vi "setSerializedData.vi"(0 "reference":refnum<class "StateTransitionEdge.lvclass">, 1 "startNode":refnum<class "AbstractNode.lvclass">, 2 "endNode":refnum<class "AbstractNode.lvclass">, 3 "xmlOut":string, 5 "error in (no error)":errorcluster) -> (14 "reference out":refnum<class "StateTransitionEdge.lvclass">, 19 "error out":errorcluster)   [LabVIEW 2014, in "StateTransitionEdge.lvclass"]
doc: "setSerializedData"
uses:
  <resource>/Framework/Providers/Open_GDS/UML/StateTransitionEdge_class/StateTransitionEdge.lvclass
  <resource>/Framework/Providers/Open_GDS/UML/AbstractNode_class/AbstractNode.lvclass
  <resource>/Framework/Providers/Open_GDS/UML/AbstractNode_class/ObjectReference.ctl
  <resource>/Framework/Providers/Open_GDS/UML/LineStyle_class/ObjectReference.ctl
  <resource>/Framework/Providers/Open_GDS/UML/ArrowHead_class/ObjectReference.ctl
  <resource>/Framework/Providers/Open_GDS/UML/General/Point/Point Point2D.ctl
  <resource>/Framework/Providers/Open_GDS/UML/BentStyle_class/ObjectReference.ctl
  <resource>/Framework/Providers/Open_GDS/UML/ReversedEngineering/ReversedEngineering_ViDependencyDetailsType.ctl
  <resource>/Framework/Providers/Open_GDS/UML/LineStyle_class/LineStyleType.ctl
  <resource>/Framework/Providers/Open_GDS/UML/ArrowHead_class/ArrowHeadType.ctl
  <resource>/Framework/Providers/Open_GDS/UML/LineStyle_class/LineStyle.lvclass
  <resource>/Framework/Providers/Open_GDS/UML/ArrowHead_class/ArrowHead.lvclass
  <resource>/Framework/Providers/Open_GDS/UML/BentStyle_class/BentStyle.lvclass
  <resource>/Framework/Providers/Open_GDS/UML/ClassRelationshipEdge_class/ClassRelationshipEdge.lvclass
  <resource>/Framework/Providers/Open_GDS/UML/SegmentedLineEdge_class/SegmentedLineEdge.lvclass
  <resource>/Framework/Providers/Open_GDS/UML/AbstractEdge_class/AbstractEdge.lvclass
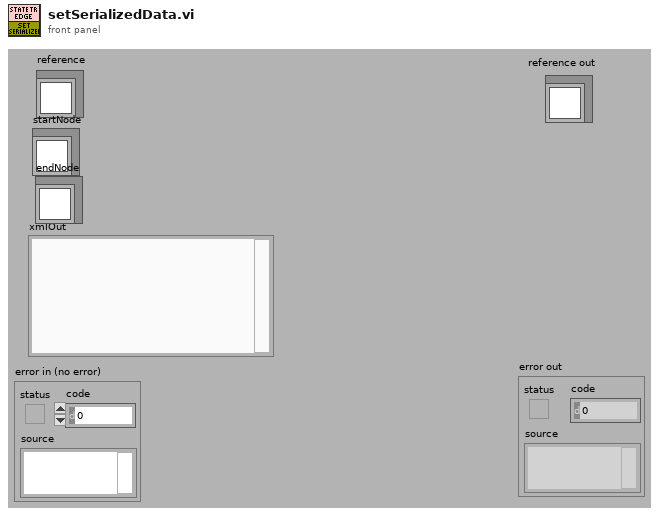
[diagram p1: front panel]
types:
  T1 = typedef "LineStyle.lvclass/ObjectReference.ctl" = refnum<k1>
  T2 = typedef "ArrowHead.lvclass/ObjectReference.ctl" = refnum<k1>
  T3 = typedef "Point Point2D.ctl" = cluster{"x":dbl, "y":dbl}
  T4 = typedef "BentStyle.lvclass/ObjectReference.ctl" = refnum<k1>
  T5 = typedef "ReversedEngineering_ViDependencyDetailsType.ctl" = cluster{"ThisVIs/Ctls":path[], "Dependent_VIs/Ctls":path[]}
  T6 = typedef "AbstractNode.lvclass/ObjectReference.ctl" = refnum<k1>
  T7 = cluster{"Base class":cluster{"Base class":cluster{"Base class":cluster{"Base class":cluster{"start":T6, "end":T6}}, "lineStyle":T1, "startArrowHead":T2, "endArrowHead":T2, "startLabel":string, "midLabel":string, "endLabel":string, "MidLabelOffset":T3, "SplitWire":bool}, "bentStyleRef":T4, "startConnectionOffset":cluster{"x":i32, "y":i32}, "endConnectionOffset":cluster{"x":i32, "y":i32}, "MidLineOffset":cluster{"x":i32, "y":i32}, "DepClass":T5}, "angle":dbl}
  T8 = typedef "LineStyle.lvclass/LineStyleType.ctl" = enum16{"SOLID", "DOTTED"}
  T9 = typedef "ArrowHead.lvclass/ArrowHeadType.ctl" = enum16{"NONE", "TRIANGLE", "BLACK_TRIANGLE", "V", "HALF_V", "DIAMOND", "BLACK_DIAMOND"}
  T10 = cluster{"Attributes":cluster{"Base class":cluster{"Base class":cluster{"Base class":cluster{"Base class":cluster{"start":T6, "end":T6}}, "lineStyle":T1, "startArrowHead":T2, "endArrowHead":T2, "startLabel":string, "midLabel":string, "endLabel":string, "MidLabelOffset":T3, "SplitWire":bool}, "bentStyleRef":T4, "startConnectionOffset":cluster{"x":i32, "y":i32}, "endConnectionOffset":cluster{"x":i32, "y":i32}, "MidLineOffset":cluster{"x":i32, "y":i32}, "DepClass":T5}, "angle":dbl}, string, string, string}
  T11 = typedef "SegmentedLineEdge.lvclass/ObjectAttributes.ctl" = cluster{"lineStyle":refnum<class "LineStyle.lvclass">, "startArrowHead":refnum<class "ArrowHead.lvclass">, "endArrowHead":refnum<class "ArrowHead.lvclass">, "startLabel":string, "midLabel":string, "endLabel":string, "MidLabelOffset":T3, "SplitWire":bool}
  T12 = typedef "AbstractEdge.lvclass/ObjectAttributes.ctl" = cluster{"start":refnum<class "AbstractNode.lvclass">, "end":refnum<class "AbstractNode.lvclass">}
  T13 = typedef "StateTransitionEdge.lvclass/ObjectAttributes.ctl" = cluster{"angle":dbl}
  T14 = typedef "ClassRelationshipEdge.lvclass/ObjectAttributes.ctl" = cluster{"bentStyleRef":refnum<class "BentStyle.lvclass">, "startConnectionOffset":cluster{"x":i32, "y":i32}, "endConnectionOffset":cluster{"x":i32, "y":i32}, "MidLineOffset":cluster{"x":i32, "y":i32}, "DepClass":T5}
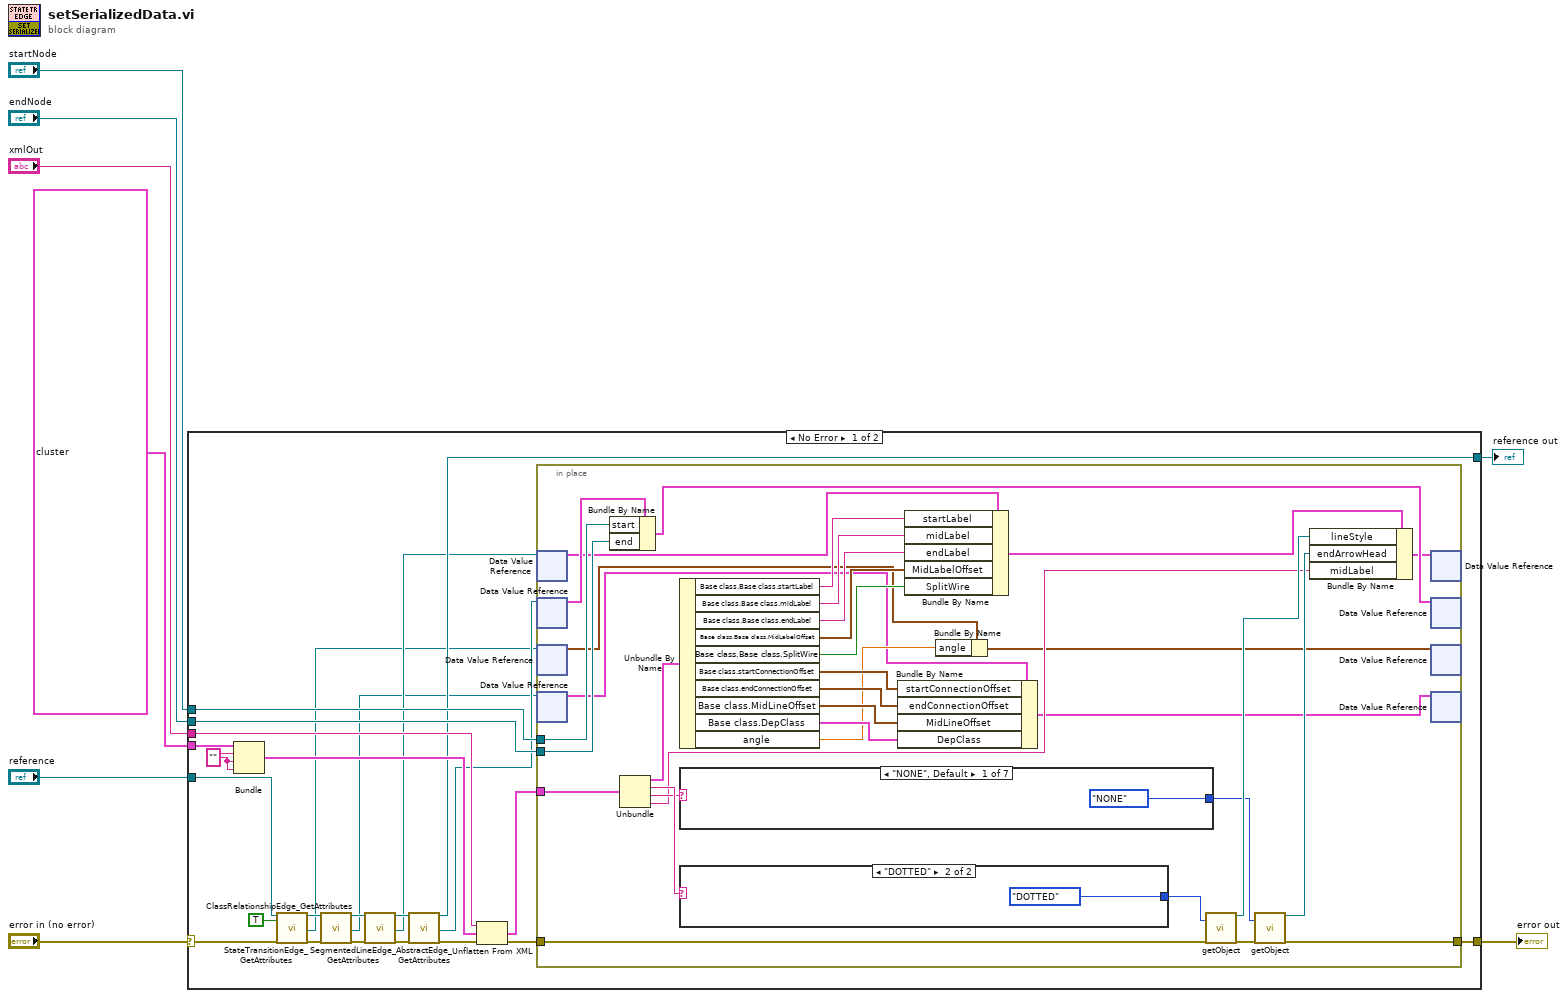
[diagram p0: block diagram]
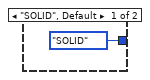
[diagram p2: hidden frame]
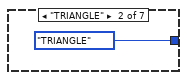
[diagram p3: hidden frame]
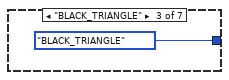
[diagram p4: hidden frame]
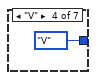
[diagram p5: hidden frame]
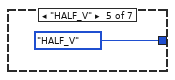
[diagram p6: hidden frame]
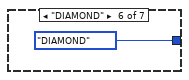
[diagram p7: hidden frame]
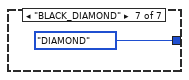
[diagram p8: hidden frame]
diagram:
  n1 = case shown="No Error" "error in (no error)" {
    selector: "error in (no error)" -> [w31 w75]
    tunnel: "reference" -> [w32 w76]
    tunnel: [w13 w76] -> w6
    tunnel: [w30 w75] -> w5
    tunnel: "xmlOut" -> [w19 _]
    tunnel: "startNode" -> [w29 _]
    tunnel: "endNode" -> [w28 _]
    tunnel: T7 {"Base class"={"Base class"={"Base class"={"Base class"={"start"=refnum, "end"=refnum}}, "lineStyle"=refnum, "startArrowHead"=refnum, "endArrowHead"=refnum, "startLabel"="", "midLabel"="", "endLabel"="", "MidLabelOffset"={"x"=0.0, "y"=0.0}, "SplitWire"=FALSE}, "bentStyleRef"=refnum, "startConnectionOffset"={"x"=0, "y"=0}, "endConnectionOffset"={"x"=0, "y"=0}, "MidLineOffset"={"x"=0, "y"=0}, "DepClass"={"ThisVIs/Ctls"=[], "Dependent_VIs/Ctls"=[]}}, "angle"=0.0} ("Attributes") -> [w26 _]
    frame No Error {
      w27 = ""
      n2 = Bundle("Attributes"=w26, w27, w27, w27) -> (w17:T10)  [unwired: 1 out]
      n3 = call <resource>:"StateTransitionEdge_GetAttributes.vi"("reference in"=w32, "OnlyGetDvrReference(False)"=TRUE, "error in (no error)"=w31) -> ("reference out"=w24:refnum<class "StateTransitionEdge.lvclass">, "DataRef"=w9:refnum<data-value>, "error out"=w23:errorcluster)  [unwired: 13 in, 1 out]
      n4 = call <resource>:"ClassRelationshipEdge_GetAttributes.vi"("reference in"=w24, "error in (no error)"=w23) -> ("reference out"=w22:refnum<class "StateTransitionEdge.lvclass">, "DataRef"=w10:refnum<data-value>, "error out"=w21:errorcluster)  [unwired: 14 in, 1 out]
      n5 = call <resource>:"SegmentedLineEdge_GetAttributes.vi"("reference in"=w22, "error in (no error)"=w21) -> ("reference out"=w16:refnum<class "StateTransitionEdge.lvclass">, "DataRef"=w11:refnum<data-value>, "error out"=w15:errorcluster)  [unwired: 14 in, 1 out]
      n6 = call <resource>:"AbstractEdge_GetAttributes.vi"("reference in"=w16, "error in (no error)"=w15) -> ("reference out"=w13:refnum<class "StateTransitionEdge.lvclass">, "DataRef"=w12:refnum<data-value>, "error out"=w14:errorcluster)  [unwired: 14 in, 1 out]
      n7 = Unflatten From XML(xml string=w19, type=w17, error in (no error)=w14) -> (value=w20:T10, error out=w18:errorcluster)
      n8 = in-place {
        in-place-border: [w63] -> w30
        in-place-border: w29 -> [w43]
        in-place-border: w28 -> [w42]
        in-place-border: w20 -> [w59]
        in-place-border: w18 -> [w58]
        n9 = in-place-dvr #1(w11) -> (w39:T11)  [unwired: 1 out]
        n10 = in-place-dvr #2(w12) -> (w41:T12)  [unwired: 1 out]
        n11 = in-place-dvr #3(w9) -> (w35:T13)  [unwired: 1 out]
        n12 = in-place-dvr #4(w10) -> (w36:T14)  [unwired: 1 out]
        n13 = Bundle By Name(cluster=w41, "start"=w43, "end"=w42) -> (w40:T12)
        n14 = Unbundle(w59) -> ("Attributes"=w47:T7, w46:string, w45:string, w44:string)
        n15 = Unbundle By Name(w47) -> ("Base class.Base class.startLabel"=w57:string, "Base class.Base class.midLabel"=w56:string, "Base class.Base class.endLabel"=w55:string, "Base class.Base class.MidLabelOffset"=w54:T3, "Base class.Base class.SplitWire"=w53:bool, "Base class.startConnectionOffset"=w52:cluster{"x":i32, "y":i32}, "Base class.endConnectionOffset"=w51:cluster{"x":i32, "y":i32}, "Base class.MidLineOffset"=w50:cluster{"x":i32, "y":i32}, "Base class.DepClass"=w49:T5, "angle"=w48:dbl)
        n16 = case shown="\"NONE\", Default" w45 {
          tunnel: [ArrowHeadType."NONE" ("arrowHead") ArrowHeadType."TRIANGLE" ("arrowHead") ArrowHeadType."BLACK_TRIANGLE" ("arrowHead") ArrowHeadType."V" ("arrowHead") ArrowHeadType."HALF_V" ("arrowHead") ArrowHeadType."DIAMOND" ("arrowHead") ArrowHeadType."DIAMOND" ("arrowHead")] -> w62
          frame "NONE", Default {
          }
          frame "TRIANGLE" {
          }
          frame "BLACK_TRIANGLE" {
          }
          frame "V" {
          }
          frame "HALF_V" {
          }
          frame "DIAMOND" {
          }
          frame "BLACK_DIAMOND" {
          }
        }
        n17 = case shown="\"DOTTED\"" w46 {
          tunnel: [LineStyleType."SOLID" ("lineStyle") LineStyleType."DOTTED" ("lineStyle")] -> w60
          frame "SOLID", Default {
          }
          frame "DOTTED" {
          }
        }
        n18 = Bundle By Name(cluster=w36, "startConnectionOffset"=w52, "endConnectionOffset"=w51, "MidLineOffset"=w50, "DepClass"=w49) -> (w33:T14)
        n19 = Bundle By Name(cluster=w39, "startLabel"=w57, "midLabel"=w56, "endLabel"=w55, "MidLabelOffset"=w54, "SplitWire"=w53) -> (w38:T11)
        n20 = Bundle By Name(cluster=w35, "angle"=w48) -> (w34:T13)
        n21 = call <resource>:"getObject.vi"("lineStyle"=w60, "error in (no error)"=w58) -> ("reference out"=w65:refnum<class "LineStyle.lvclass">, "error out"=w61:errorcluster)  [unwired: 16 out]
        n22 = call <resource>:"getObject.vi"("arrowHead"=w62, "error in (no error)"=w61) -> ("reference out"=w64:refnum<class "ArrowHead.lvclass">, "error out"=w63:errorcluster)  [unwired: 16 out]
        n23 = Bundle By Name(cluster=w38, "lineStyle"=w65, "endArrowHead"=w64, "midLabel"=w44) -> (w37:T11)
        n24 = in-place-dvr #1(w37) -> ()  [unwired: 2 out]
        n25 = in-place-dvr #2(w40) -> ()  [unwired: 2 out]
        n26 = in-place-dvr #3(w34) -> ()  [unwired: 2 out]
        n27 = in-place-dvr #4(w33) -> ()  [unwired: 2 out]
      }
    }
    frame Error {
    }
  }
  "reference out" <- w6
  "error out" <- w5
